vi "TemperatureControl_CuiLab.vi"() -> ()   [LabVIEW 2017]
uses:
  <vilib>/Utility/file.llb/Write To Spreadsheet File (string).vi
  <instrlib>/Lake Shore 335/Public/Data/Sensor Data (Single Reading).vi
  <vilib>/Analysis/NI_AALPro.lvlib
panel:
  in  "Interval":dbl=5.0 caption="Every" format="%#_g s"
  in  "TimeStamp":dbl[](array[numeric])
  in  "T history":dbl[][](array[numeric])
  in  "Set PID":bool
  in  "Sample Temp":enum16{"A", "B", "C", "D"}(ring)
  in  "Write to File":bool
  in  "Interval (ms)":i32=500
  in  "Temperature Log File":path
  out "Temperature":T1(graph)
  out "Temp D":dbl=11.245 caption="D:"
  out "Temp C":dbl=4.276 caption="C:"
  out "Standalone":bool=TRUE
  in  "Set":bool
  in  "Refresh":bool
  in  "Manual Output (%)":dbl
  in  "Loop 1 Heater Range":u16(ring)=3 items=["Off", "Low (0.5W)", "Med (5W)", "High (50W)"]
  in  "Rate (D)":dbl=20.0
  in  "Reset (I)":dbl=10.0
  in  "Gain (P)":dbl=10.0
  in  "Ramp Rate (K/min)":dbl=10.0
  in  "Ramp":bool=TRUE
  in  "Setpoint (K)":dbl=4.0
  in  "Quit":bool
  in  "Loop":u16(ring) items=["1"=1, "2"=2]
  in  "Model":enum16{"LS 335", "LS 340"}(ring)
  in  "VISA resource name":refnum<visa-resource-name>="Lakeshore"
  in  "Connect":bool
  out "Heater Output":dbl(slide) scale=0.0..100.0
  out "Heater Range Status":string="High"
  out "Setpoint status":dbl=4.0 caption="S:"
  out "Temp B":dbl=11.245 caption="B:"
  out "Temp A":dbl=4.276 caption="A:"
  # "Rates (K/min)"
  # "K"
  # "K"
  # "K"
  # "K"
  # "K"
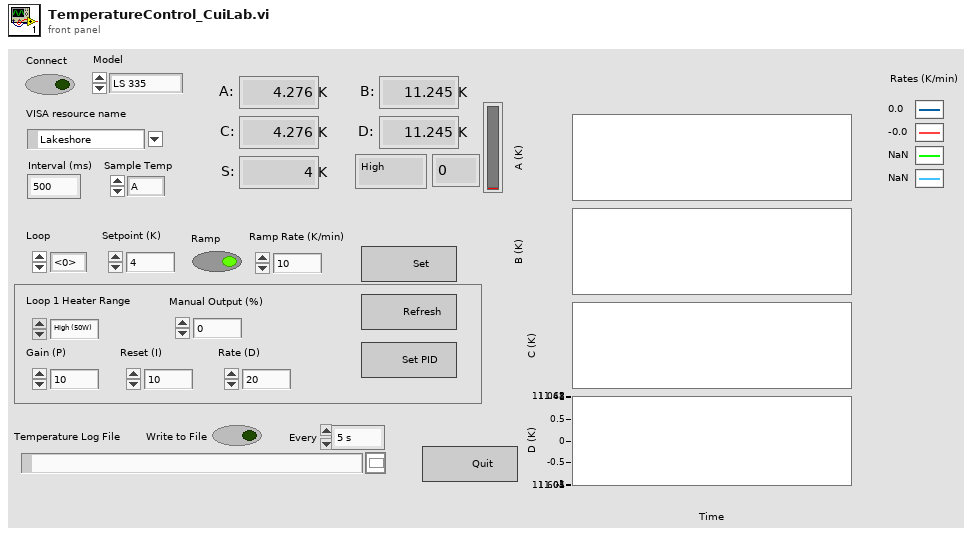
[diagram p1: front panel]
types:
  T1 = cluster{"[0]":dbl, "[1]":dbl, "[2]":dbl, "[3]":dbl}
  T2 = enum16{"Init", "Read", "ScannerVXY", "ScannerVZ", "ScannerVXYZ", "Temp", "Field", "He", "Encoder", "MIM", "NanonisMon", "ScannerXYZ"}
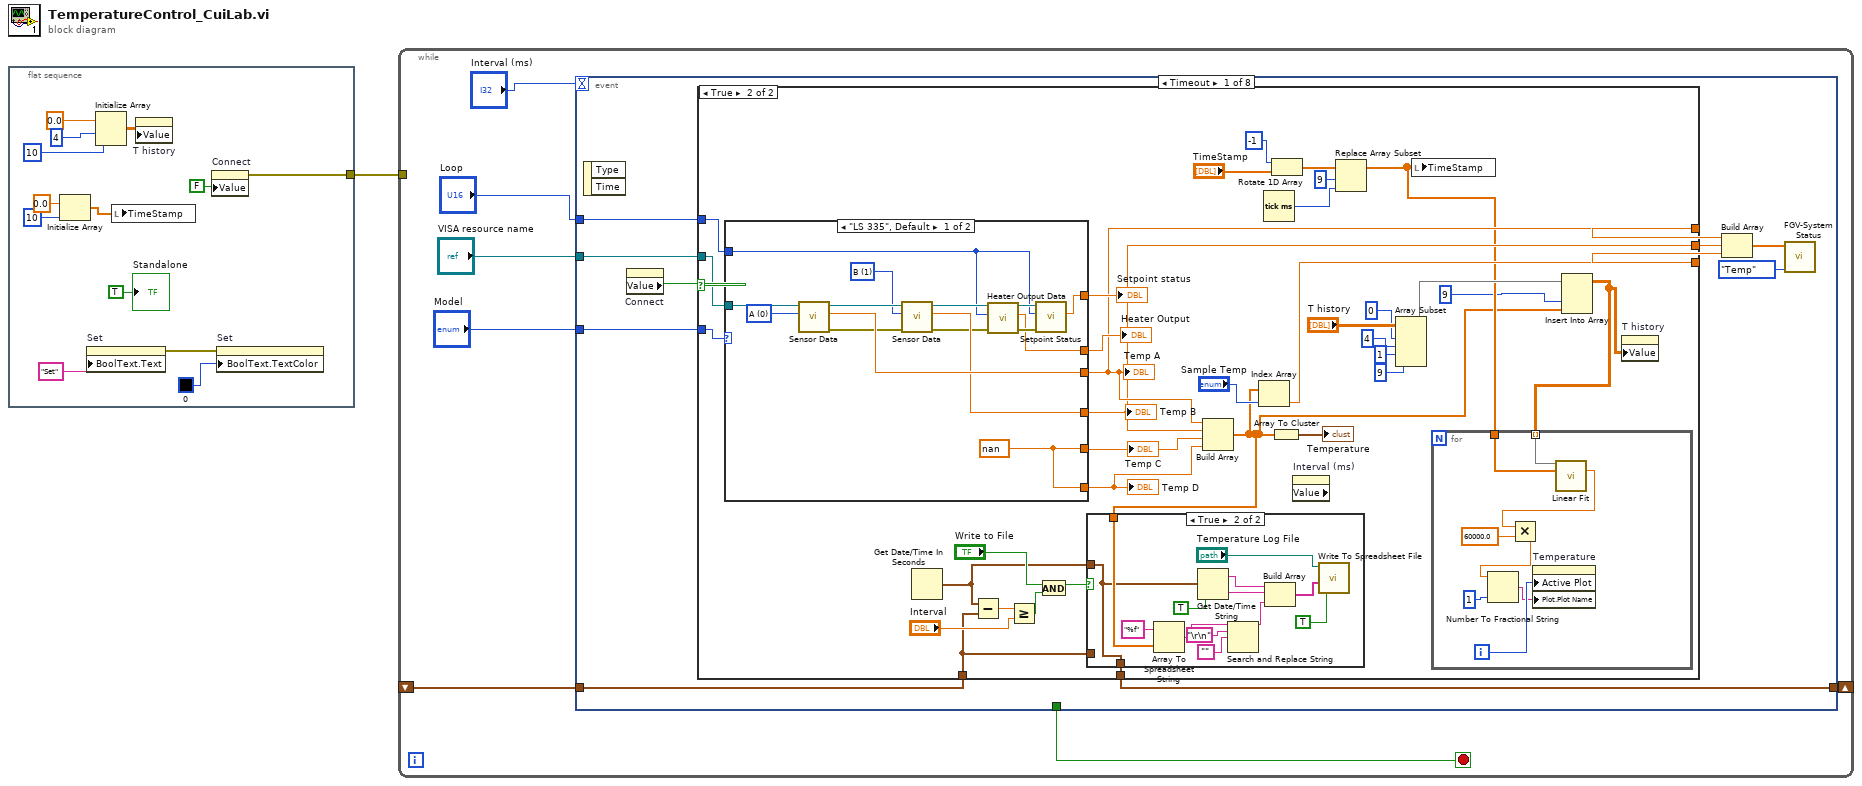
[diagram p0: block diagram]
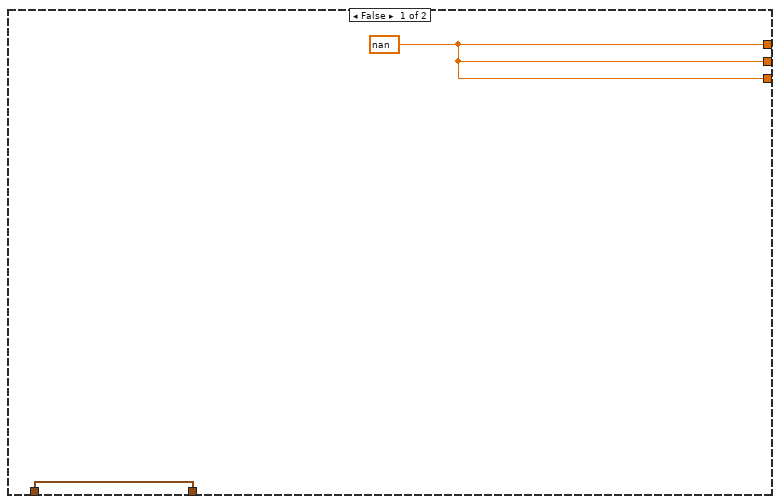
[diagram p2: hidden frame]
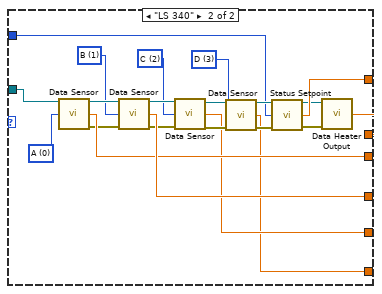
[diagram p4: hidden frame]
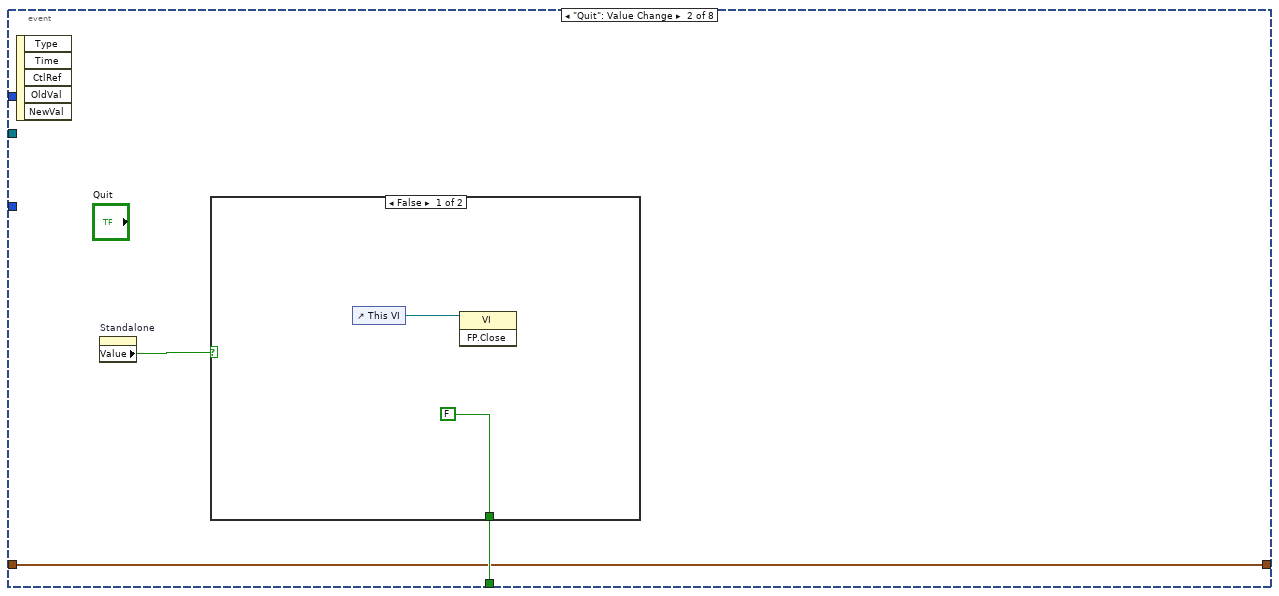
[diagram p5: hidden frame]
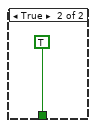
[diagram p6: hidden frame]
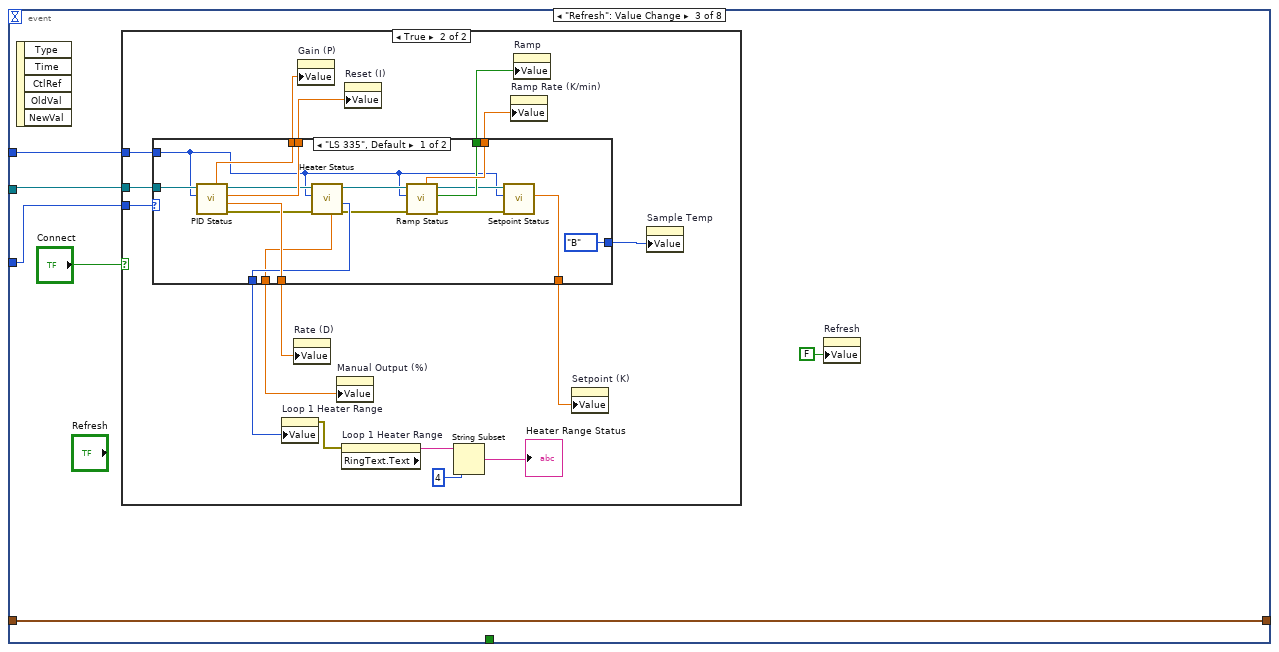
[diagram p7: hidden frame]
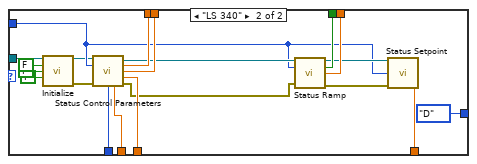
[diagram p9: hidden frame]
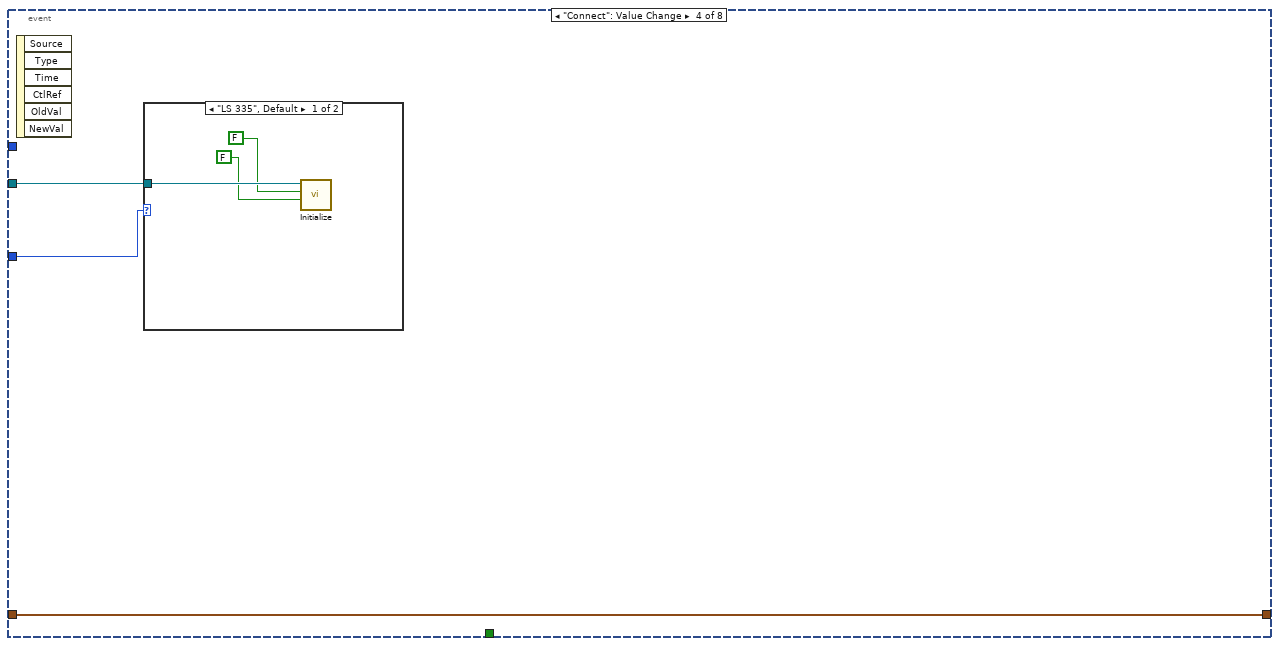
[diagram p10: hidden frame]
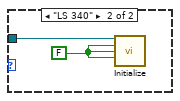
[diagram p11: hidden frame]
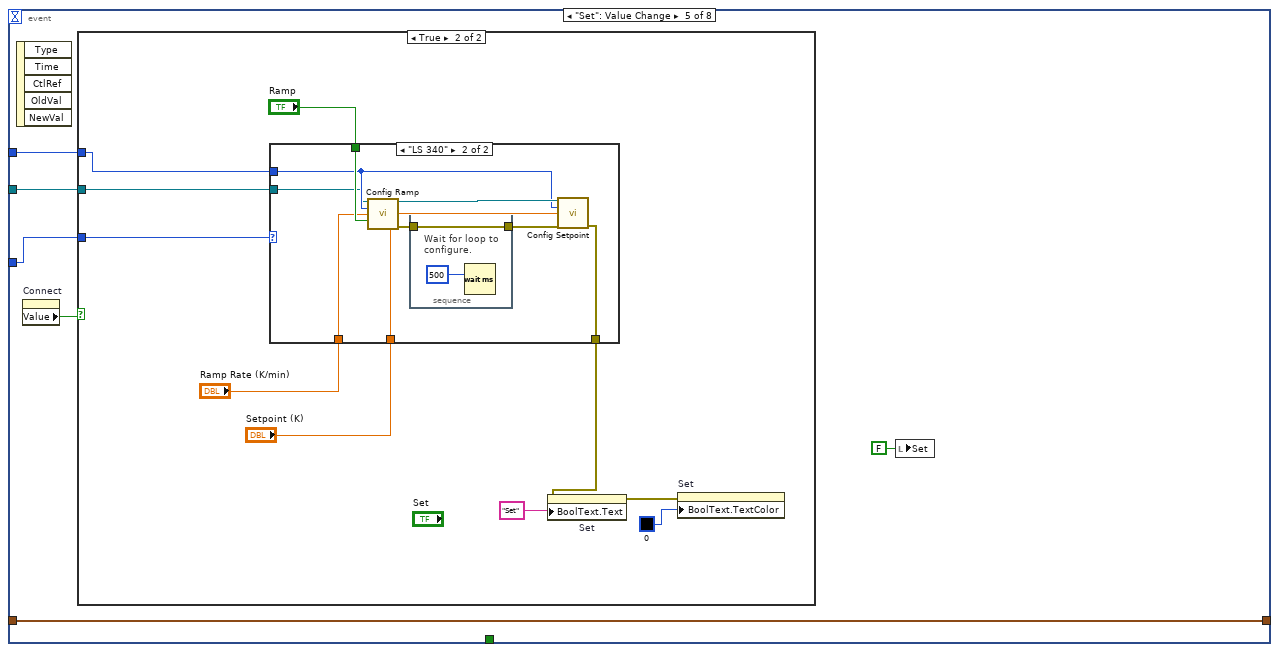
[diagram p12: hidden frame]
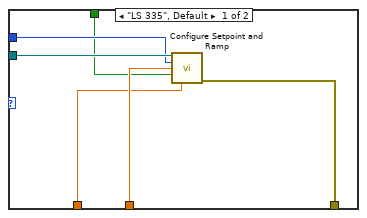
[diagram p14: hidden frame]
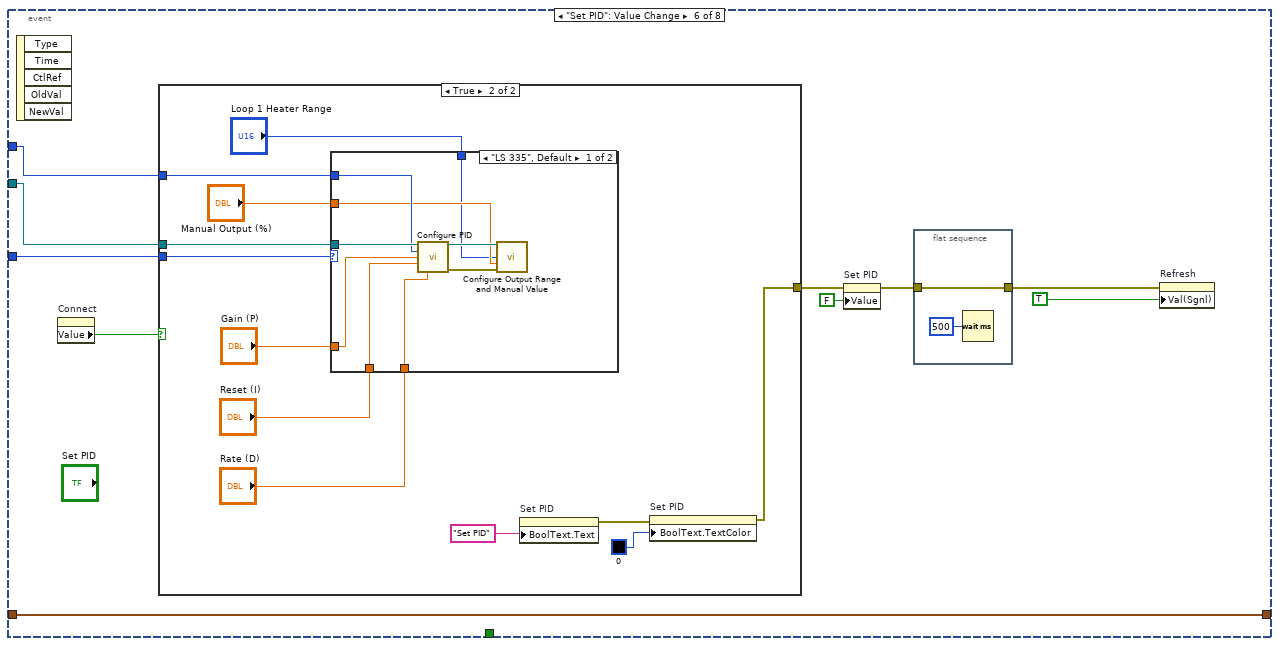
[diagram p15: hidden frame]
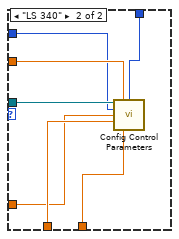
[diagram p17: hidden frame]
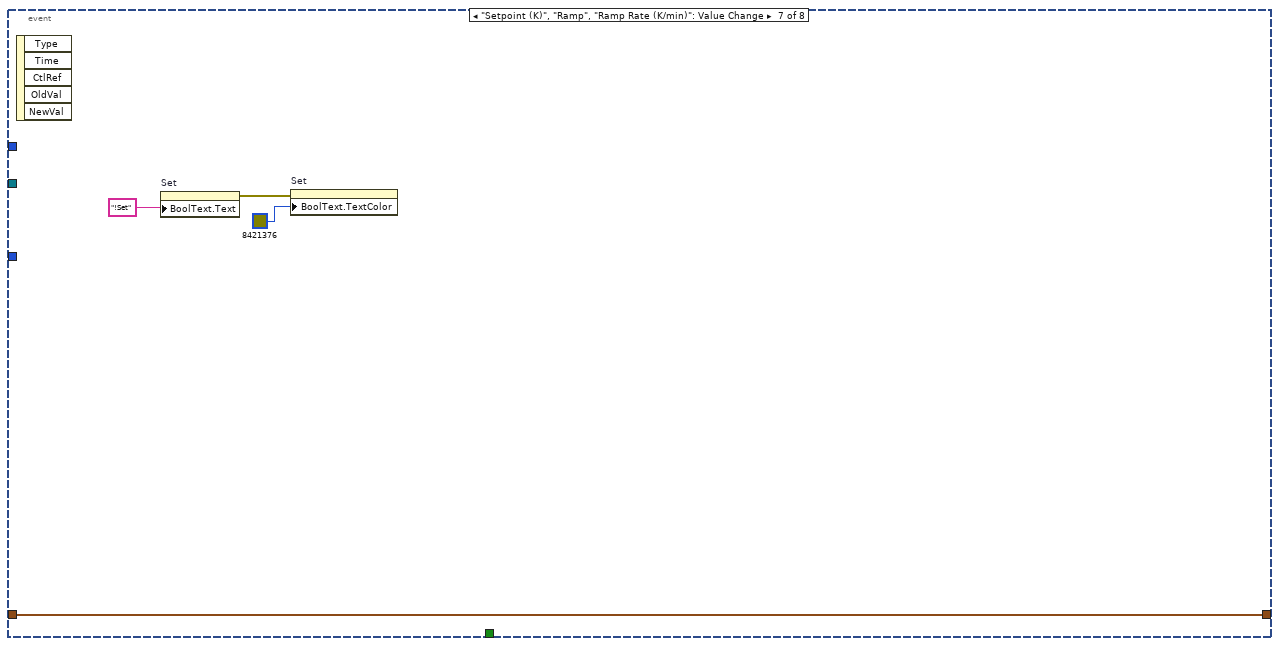
[diagram p18: hidden frame]
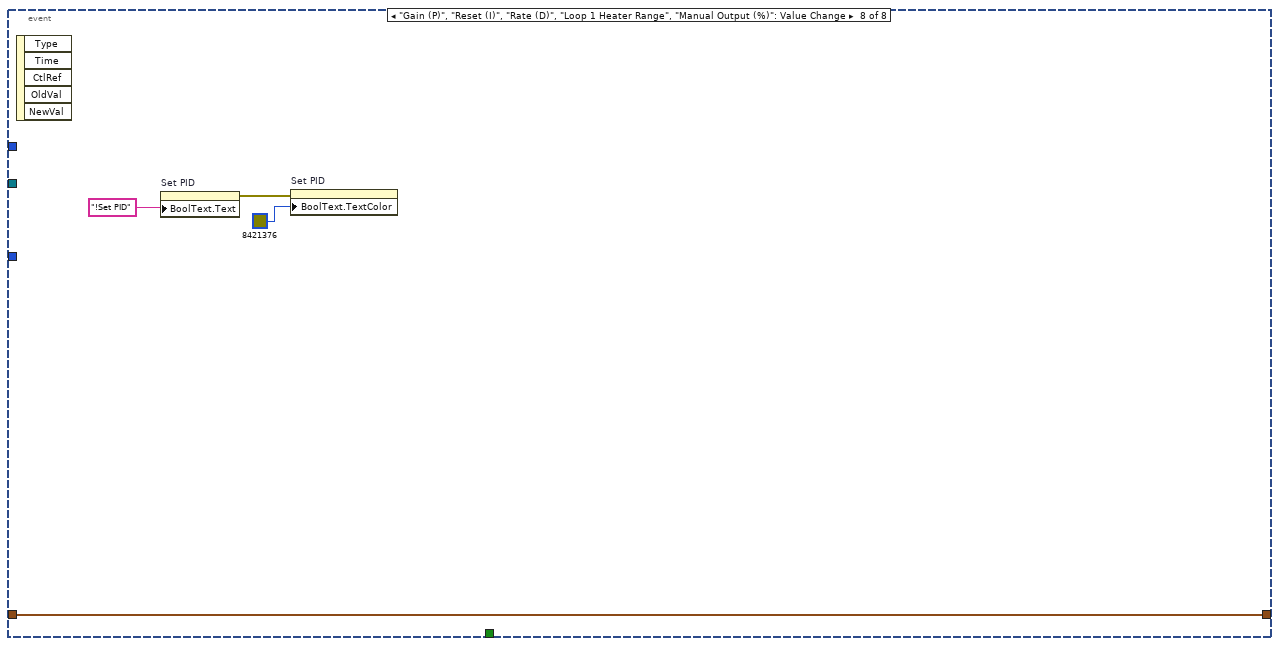
[diagram p19: hidden frame]
diagram:
  n1 = flat-sequence {
    tunnel: [w13] -> w1
    frame #0 {
      n2 = Initialize Array(0.0 ("element"), 10 ("dimension size")) -> (w2:dbl[])
      n3 = property on="Set" class="Bool (strict)"("BoolText.Text"="Set" ("Label.Text")) -> (error out=w10:errorcluster)  [unwired: 2 in, 1 out]
      n4 = Initialize Array(0.0 ("element"), 4 ("dimension size"), 10 ("dimension size")) -> (w6:dbl[][])
      n5 = local write "TimeStamp"(w2) -> ()
      n6 = property on="T history" class="Arr (strict)"("Value"=w6) -> ()  [unwired: 2 in, 2 out]
      n7 = property on="Connect" class="Bool (strict)"("Value"=FALSE ("Connect")) -> (error out=w13:errorcluster)  [unwired: 2 in, 1 out]
      n8 = property on="Set" class="Bool (strict)"(error in=w10, "BoolText.TextColor"=u32 0) -> ()  [unwired: 1 in, 2 out]
      "Standalone" <- TRUE ("Standalone")
    }
  }
  n9 = while {
    tunnel: w1 -> [_]
    shift-right: [w16] -> _
    shift-left: _ -> [w15]
    stop <- w18 stop-if-true
    n10 = event shown="[0] Timeout" {
      selector: _ -> [_ _ _ _ _ _ _ _]
      dyn-events: _ -> [_ _ _ _ _ _ _ _]
      timeout: "Interval (ms)" -> [_ _ _ _ _ _ _ _]
      tunnel: "VISA resource name" -> [w32 _ w140 w196 w207 w242 _ _]
      tunnel: "Model" -> [w31 _ w138 w195 w205 w243 _ _]
      tunnel: "Loop" -> [w30 _ w139 _ w206 w241 _ _]
      tunnel: [_ w130 _ _ _ _ _ _] -> w18
      tunnel: [w23 w129 w135 w194 w202 w235 w275 w279] -> w16
      tunnel: w15 -> [w22 w129 w135 w194 w202 w235 w275 w279]
      event Timeout {
        n11 = event-data() -> ()  [unwired: 1 in, 2 out]
        n12 = property on="Connect" class="Bool (strict)"() -> ("Value"=w29:bool)  [unwired: 2 in, 2 out]
        n13 = case shown="True" w29 {
          tunnel: w32 -> [_ w69]
          tunnel: w31 -> [_ w68]
          tunnel: w30 -> [_ w67]
          tunnel: [w34 w59] -> w28
          tunnel: [w34 w58] -> w27
          tunnel: [w34 w57] -> w26
          tunnel: [w33 w44] -> w23
          tunnel: w22 -> [w33 w38]
          frame False {
            w34 = nan ("Kelvin Reading")
          }
          frame True {
            n14 = case shown="\"LS 335\", Default" w68 {
              tunnel: w69 -> [w105 w128]
              tunnel: [w103 w123] -> w59
              tunnel: [w100 w124] -> w58
              tunnel: [w96 w122] -> w66
              tunnel: [w92 w119] -> w65
              tunnel: [w106 w109] -> w62
              tunnel: [w106 w108] -> w61
              tunnel: w67 -> [w94 w107]
              frame "LS 335", Default {
                w101 = u16 1 items=["A", "B"] ("Input (0:A)")
                w104 = u16 0 items=["A", "B"] ("Input (0:A)")
                w106 = nan ("Kelvin Reading")
                n15 = call-poly <instrlib>:"Sensor Data.vi"("Input (0:A)"=w104, "VISA resource name"=w105) -> ("error out"=w98:errorcluster, "Sensor Data"=w103:dbl, "VISA resource name out"=w102:refnum<visa-resource-name>)  [unwired: 7 in]
                n16 = call-poly <instrlib>:"Sensor Data.vi"("error in (no error)"=w98, "Input (0:A)"=w101, "VISA resource name"=w102) -> ("error out"=w97:errorcluster, "Sensor Data"=w100:dbl, "VISA resource name out"=w99:refnum<visa-resource-name>)  [unwired: 6 in]
                n17 = call <instrlib>:"Heater Output Data.vi"("error in (no error)"=w97, "Heater Output (1:1)"=w94, "VISA resource name"=w99) -> ("error out"=w93:errorcluster, "Output Value"=w92:dbl, "VISA resource name out"=w95:refnum<visa-resource-name>)  [unwired: 6 in]
                n18 = call <instrlib>:"Setpoint Status.vi"("error in (no error)"=w93, "Output (1:1)"=w94, "VISA resource name"=w95) -> ("Setpoint"=w96:dbl)  [unwired: 6 in, 2 out]
              }
              frame "LS 340" {
                w110 = u16 3 items=["A", "B", "C", "D"] ("Input (0: A)")
                w111 = u16 2 items=["A", "B", "C", "D"] ("Input (0: A)")
                w125 = u16 1 items=["A", "B", "C", "D"] ("Input (0: A)")
                w127 = u16 0 items=["A", "B", "C", "D"] ("Input (0: A)")
                n19 = call <instrlib>:"Data Sensor.vi"("VISA resource name"=w128, "Input (0: A)"=w127) -> ("VISA resource name out"=w126:refnum<visa-resource-name>, "Kelvin Reading"=w123:dbl, "error out"=w118:errorcluster)  [unwired: 9 in, 2 out]
                n20 = call <instrlib>:"Data Sensor.vi"("VISA resource name"=w126, "Input (0: A)"=w125, "error in (no error)"=w118) -> ("VISA resource name out"=w117:refnum<visa-resource-name>, "Kelvin Reading"=w124:dbl, "error out"=w116:errorcluster)  [unwired: 8 in, 2 out]
                n21 = call <instrlib>:"Data Sensor.vi"("VISA resource name"=w117, "Input (0: A)"=w111, "error in (no error)"=w116) -> ("VISA resource name out"=w115:refnum<visa-resource-name>, "Kelvin Reading"=w109:dbl, "error out"=w112:errorcluster)  [unwired: 8 in, 2 out]
                n22 = call <instrlib>:"Data Sensor.vi"("VISA resource name"=w115, "Input (0: A)"=w110, "error in (no error)"=w112) -> ("VISA resource name out"=w114:refnum<visa-resource-name>, "Kelvin Reading"=w108:dbl, "error out"=w113:errorcluster)  [unwired: 8 in, 2 out]
                n23 = call <instrlib>:"Status Setpoint.vi"("VISA resource name"=w114, "Loop (0: 1)"=w107, "error in (no error)"=w113) -> ("VISA resource name out"=w121:refnum<visa-resource-name>, "Setpoint"=w122:dbl, "error out"=w120:errorcluster)  [unwired: 10 in]
                n24 = call <instrlib>:"Data Heater Output.vi"("VISA resource name"=w121, "error in (no error)"=w120) -> ("Heater Output"=w119:dbl)  [unwired: 11 in, 2 out]
              }
            }
            "Temp A" <- w59
            "Temp B" <- w58
            "Setpoint status" <- w66
            "Heater Output" <- w65
            "Temp D" <- w61
            "Temp C" <- w62
            n25 = Get Date/Time In Seconds() -> (seconds since 1Jan1904=w43:timestamp)
            n26 = Subtract(x=w43, y=w38) -> (x-y=w42:dbl)
            n27 = Greater Or Equal?(x=w42, y="Interval") -> (x >= y?=w39:bool)
            n28 = And(x="Write to File", y=w39) -> (x .and. y?=w40:bool)
            n29 = Build Array(w59, w58, w62, w61) -> (w37:dbl[])
            n30 = case shown="True" w40 {
              tunnel: w37 -> [_ w84]
              tunnel: [w78 w79] -> w44
              tunnel: w43 -> [_ w79]
              tunnel: w38 -> [w78 _]
              frame False {
              }
              frame True {
                n31 = Array To Spreadsheet String(array=w84, 3:"%f" ("format string")) -> (spreadsheet string=w82:string)  [unwired: 1 in]
                n32 = Get Date/Time String(seconds (now)=w79, want seconds? (F)=TRUE) -> (date string=w90:string, time string=w89:string)  [unwired: 1 in]
                n33 = Search and Replace String(input string=w82, search string="\r\n", replace string="") -> (result string=w83:string)  [unwired: 5 in, 3 out]
                n34 = Build Array(w90, w89, w83) -> (w87:string[])
                n35 = call-poly <vilib>:"Write To Spreadsheet File.vi"("append to file? (new file:F)"=TRUE, "1D data"=w87, "file path (dialog if empty)"="Temperature Log File") -> ()  [unwired: 5 in, 1 out]
              }
            }
            n36 = Index Array(array=w37, index="Sample Temp") -> (element=w57:dbl)
            n37 = Tick Count (ms)() -> (millisecond timer value=w46:u32)
            n38 = Array To Cluster(array=w37) -> (cluster=→"Temperature":T1)
            n39 = Rotate 1D Array(1:"TimeStamp", 2:-1 ("n")) -> (0:w48:dbl[])
            n40 = property on="Interval (ms)" class="DigNum (strict)" props=["Value"]() -> ()  [unwired: 2 in, 3 out]
            n41 = Replace Array Subset(array=w48, new element=w46, index=9) -> (w45:dbl[])
            n42 = Array Subset(array="T history", index (row)=0 ("index"), length (row)=4 ("length"), index (col)=1 ("index"), length (col)=9 ("length")) -> (w51:dbl[][])
            n43 = local write "TimeStamp"(w45) -> ()
            n44 = Insert Into Array(array=w51, index (col)=9 ("disabled index (col)"), new element=w37) -> (w36:dbl[][])  [unwired: 1 in]
            n45 = for {
              tunnel: w45 -> [w73]
              tunnel: w36 -> [w70] mode=indexing
              i -> [w77]
              n46 = call <vilib>:"Linear Fit.vi"("Y"=w70, "X"=w73) -> ("slope"=w71:dbl)  [unwired: 9 in, 4 out]
              n47 = Multiply(x=w71, y=60000.0) -> (x*y=w76:dbl)
              n48 = Number To Fractional String(number=w76, precision (6)=i16 1) -> (F-format string=w74:string)  [unwired: 2 in]
              n49 = property on="Temperature" class="WFChart (strict)"("Active Plot"=w77, "Plot.Plot Name"=w74) -> ()  [unwired: 2 in, 2 out]
            }
            n50 = property on="T history" class="Arr (strict)"("Value"=w36) -> ()  [unwired: 2 in, 2 out]
          }
        }
        n51 = Build Array(w28, w27, w26) -> (w25:dbl[])
        n52 = call "FGV-System Status.vi"("Action"=T2."Temp", "Input Data"=w25) -> ()  [unwired: 9 in, 1 out]
      }
      event "Quit": Value Change {
        n53 = event-data() -> ()  [unwired: 1 in, 5 out]
        n54 = property on="Standalone" class="Bool (strict)"() -> ("Value"=w131:bool)  [unwired: 2 in, 2 out]
        n55 = case shown="False" w131 {
          tunnel: [FALSE TRUE] -> w130
          frame False {
            n56 = control-ref of="This VI"() -> (w132:refnum<vi>)
            n57 = invoke class="VI" method="FP.Close"(reference=w132) -> ()  [unwired: 2 in, 3 out]
          }
          frame True {
          }
        }
      }
      event "Refresh": Value Change {
        n58 = event-data() -> ()  [unwired: 1 in, 5 out]
        n59 = case shown="True" "Connect" {
          tunnel: w140 -> [_ w156]
          tunnel: w139 -> [_ w149]
          tunnel: w138 -> [_ w146]
          frame False {
          }
          frame True {
            n60 = case shown="\"LS 335\", Default" w146 {
              tunnel: w156 -> [w172 w178]
              tunnel: [w170 w193] -> w155
              tunnel: [w171 w192] -> w154
              tunnel: [w169 w191] -> w153
              tunnel: [w166 w190] -> w152
              tunnel: [w162 w187] -> w151
              tunnel: [w163 w186] -> w150
              tunnel: w149 -> [w159 w183]
              tunnel: [w157 w182] -> w148
              tunnel: [w167 w181] -> w147
              tunnel: [enum16{"A", "B", "C", "D"}."B" ("Sample Temp") enum16{"A", "B", "C", "D"}."D" ("Sample Temp")] -> w141
              frame "LS 335", Default {
                n61 = call <instrlib>:"PID Status.vi"("Output's Control Loop (1:1)"=w159, "VISA resource name"=w172) -> ("error out"=w165:errorcluster, "Rate (D)"=w169:dbl, "Reset (I)"=w171:dbl, "VISA resource name out"=w168:refnum<visa-resource-name>, "Gain (P)"=w170:dbl)  [unwired: 5 in]
                n62 = call <instrlib>:"Heater Status.vi"("error in (no error)"=w165, "Heater Output (1:1)"=w159, "VISA resource name"=w168) -> ("error out"=w161:errorcluster, "Heater Range"=w167:u16, "VISA resource name out"=w164:refnum<visa-resource-name>, "Manual Output Value"=w166:dbl)  [unwired: 4 in, 1 out]
                n63 = call <instrlib>:"Ramp Status.vi"("error in (no error)"=w161, "Output's Control Loop (1:1)"=w159, "VISA resource name"=w164) -> ("error out"=w158:errorcluster, "Ramping On"=w162:bool, "VISA resource name out"=w160:refnum<visa-resource-name>, "Ramp Rate"=w163:dbl)  [unwired: 4 in, 1 out]
                n64 = call <instrlib>:"Setpoint Status.vi"("error in (no error)"=w158, "Output (1:1)"=w159, "VISA resource name"=w160) -> ("Setpoint"=w157:dbl)  [unwired: 6 in, 2 out]
              }
              frame "LS 340" {
                n65 = call <instrlib>:"Initialize.vi"("VISA resource name"=w178, "ID Query (T: Check)"=FALSE, "Reset (T: Reset)"=FALSE, "Reset Defaults (F:Dont Reset)"=FALSE) -> ("VISA resource name out"=w180:refnum<visa-resource-name>, "error out"=w179:errorcluster)  [unwired: 10 in]
                n66 = call <instrlib>:"Status Control Parameters.vi"("VISA resource name"=w180, "Loop (0: 1)"=w183, "error in (no error)"=w179) -> ("VISA resource name out"=w189:refnum<visa-resource-name>, "Gain (P)"=w193:dbl, "Reset (I)"=w192:dbl, "Rate (D)"=w191:dbl, "Loop 1 Heater Range"=w181:u16, "Manual Output"=w190:dbl, "error out"=w188:errorcluster)  [unwired: 5 in, 1 out]
                n67 = call <instrlib>:"Status Ramp.vi"("VISA resource name"=w189, "Loop (0: 1)"=w183, "error in (no error)"=w188) -> ("VISA resource name out"=w185:refnum<visa-resource-name>, "Ramping On/Off"=w187:bool, "Rate Value"=w186:dbl, "error out"=w184:errorcluster)  [unwired: 8 in, 1 out]
                n68 = call <instrlib>:"Status Setpoint.vi"("VISA resource name"=w185, "Loop (0: 1)"=w183, "error in (no error)"=w184) -> ("Setpoint"=w182:dbl)  [unwired: 10 in, 2 out]
              }
            }
            n69 = property on="Loop 1 Heater Range" class="Ring (strict)"("Value"=w147) -> (error out=w145:errorcluster)  [unwired: 2 in, 1 out]
            n70 = property on="Rate (D)" class="DigNum (strict)"("Value"=w153) -> ()  [unwired: 2 in, 2 out]
            n71 = property on="Gain (P)" class="DigNum (strict)"("Value"=w155) -> ()  [unwired: 2 in, 2 out]
            n72 = property on="Manual Output (%)" class="DigNum (strict)"("Value"=w152) -> ()  [unwired: 2 in, 2 out]
            n73 = property on="Loop 1 Heater Range" class="Ring (strict)"(error in=w145) -> ("RingText.Text"=w144:string)  [unwired: 1 in, 2 out]
            n74 = property on="Reset (I)" class="DigNum (strict)"("Value"=w154) -> ()  [unwired: 2 in, 2 out]
            n75 = String Subset(string=w144, length (rest)=4 ("length (rest)")) -> (substring=→"Heater Range Status":string)  [unwired: 1 in]
            n76 = property on="Ramp Rate (K/min)" class="DigNum (strict)"("Value"=w150) -> ()  [unwired: 2 in, 2 out]
            n77 = property on="Ramp" class="Bool (strict)"("Value"=w151) -> ()  [unwired: 2 in, 2 out]
            n78 = property on="Setpoint (K)" class="DigNum (strict)"("Value"=w148) -> ()  [unwired: 2 in, 2 out]
            n79 = property on="Sample Temp" class="Enum (strict)"("Value"=w141) -> ()  [unwired: 2 in, 2 out]
          }
        }
        n80 = property on="Refresh" class="Bool (strict)"("Value"=FALSE ("Refresh")) -> ()  [unwired: 2 in, 2 out]
      }
      event "Connect": Value Change {
        n81 = event-data() -> ()  [unwired: 1 in, 6 out]
        n82 = case shown="\"LS 335\", Default" w195 {
          tunnel: w196 -> [w199 w201]
          frame "LS 335", Default {
            n83 = call <instrlib>:"Initialize.vi"("Reset (True)"=FALSE ("ID Query (True)"), "ID Query (True)"=FALSE ("Reset (True)"), "VISA resource name"=w199) -> ()  [unwired: 7 in, 2 out]
          }
          frame "LS 340" {
            w200 = FALSE ("ID Query (T: Check)")
            n84 = call <instrlib>:"Initialize.vi"("VISA resource name"=w201, "ID Query (T: Check)"=w200, "Reset (T: Reset)"=w200, "Reset Defaults (F:Dont Reset)"=w200) -> ()  [unwired: 10 in, 2 out]
          }
        }
      }
      event "Set": Value Change {
        n85 = event-data() -> ()  [unwired: 1 in, 5 out]
        n86 = property on="Connect" class="Bool (strict)"() -> ("Value"=w204:bool)  [unwired: 2 in, 2 out]
        n87 = case shown="True" w204 {
          tunnel: w207 -> [_ w210]
          tunnel: w206 -> [_ w209]
          tunnel: w205 -> [_ w208]
          frame False {
          }
          frame True {
            n88 = case shown="\"LS 340\"" w208 {
              tunnel: w210 -> [w223 w224]
              tunnel: "Ramp" -> [w220 w232]
              tunnel: "Ramp Rate (K/min)" -> [w219 w231]
              tunnel: "Setpoint (K)" -> [w221 w229]
              tunnel: [w218 w226] -> w211
              tunnel: w209 -> [w222 w225]
              frame "LS 335", Default {
                n89 = call <instrlib>:"Configure Setpoint and Ramp.vi"("VISA resource name"=w223, "Output's Control Loop (1:1)"=w222, "Setpoint (0.0000)"=w221, "Enable Setpoint Ramping (F: Off)"=w220, "Ramp Rate (0.0)"=w219) -> ("error out"=w218:errorcluster)  [unwired: 9 in, 1 out]
              }
              frame "LS 340" {
                n90 = call <instrlib>:"Config Ramp.vi"("VISA resource name"=w224, "Loop (0: 1)"=w225, "Rate Value (0.1)"=w231, "Ramping On/Off (F: Ramping Off)"=w232) -> ("VISA resource name out"=w230:refnum<visa-resource-name>, "error out"=w228:errorcluster)  [unwired: 10 in]
                n91 = stacked-sequence {
                  tunnel: w228 -> [w233]
                  tunnel: [w233] -> w227
                  frame #0 {
                    # "Wait for loop to \nconfigure."
                    n92 = Wait (ms)(milliseconds to wait=u32 500) -> ()  [unwired: 1 out]
                  }
                }
                n93 = call <instrlib>:"Config Setpoint.vi"("VISA resource name"=w230, "Loop (0: 1)"=w225, "Setpoint (0.0)"=w229, "error in (no error)"=w227) -> ("error out"=w226:errorcluster)  [unwired: 10 in, 1 out]
              }
            }
            n94 = property on="Set" class="Bool (strict)"(error in=w211, "BoolText.Text"="Set" ("Label.Text")) -> (error out=w213:errorcluster)  [unwired: 1 in, 1 out]
            n95 = property on="Set" class="Bool (strict)"(error in=w213, "BoolText.TextColor"=u32 0) -> ()  [unwired: 1 in, 2 out]
          }
        }
        n96 = local write "Set"(FALSE ("Set")) -> ()
      }
      event "Set PID": Value Change {
        n97 = event-data() -> ()  [unwired: 1 in, 5 out]
        n98 = property on="Connect" class="Bool (strict)"() -> ("Value"=w244:bool)  [unwired: 2 in, 2 out]
        n99 = case shown="True" w244 {
          tunnel: w243 -> [_ w258]
          tunnel: w242 -> [_ w257]
          tunnel: w241 -> [_ w256]
          tunnel: [_ w247] -> w238
          frame False {
          }
          frame True {
            n100 = case shown="\"LS 335\", Default" w258 {
              tunnel: w257 -> [w267 w274]
              tunnel: w256 -> [w263 w271]
              tunnel: "Loop 1 Heater Range" -> [w259 w273]
              tunnel: "Manual Output (%)" -> [w260 w272]
              tunnel: "Reset (I)" -> [w264 w269]
              tunnel: "Rate (D)" -> [w262 w270]
              tunnel: "Gain (P)" -> [w265 w268]
              frame "LS 335", Default {
                n101 = call <instrlib>:"Configure PID.vi"("VISA resource name"=w267, "Output's Control Loop (1:1)"=w263, "Gain (P) (50.0)"=w265, "Reset (I) (20.0)"=w264, "Rate (D) (0.0 %)"=w262) -> ("VISA resource name out"=w266:refnum<visa-resource-name>, "error out"=w261:errorcluster)  [unwired: 9 in]
                n102 = call <instrlib>:"Configure Output Range and Manual Value.vi"("VISA resource name"=w266, "Range (0:Off)"=w259, "Manual Output (0.00 %)"=w260, "error in (no error)"=w261) -> ()  [unwired: 10 in, 2 out]
              }
              frame "LS 340" {
                n103 = call <instrlib>:"Config Control Parameters.vi"("VISA resource name"=w274, "Manual Output (0.00)"=w272, "Heater Range (0: Off)"=w273, "Loop (0: 1)"=w271, "Gain (P) (0.0)"=w268, "Reset (I) (0.0)"=w269, "Rate (D) (0)"=w270) -> ()  [unwired: 7 in, 2 out]
              }
            }
            n104 = property on="Set PID" class="Bool (strict)"("BoolText.Text"="Set PID" ("Label.Text")) -> (error out=w249:errorcluster)  [unwired: 2 in, 1 out]
            n105 = property on="Set PID" class="Bool (strict)"(error in=w249, "BoolText.TextColor"=u32 0) -> (error out=w247:errorcluster)  [unwired: 1 in, 1 out]
          }
        }
        n106 = property on="Set PID" class="Bool (strict)"(error in=w238, "Value"=FALSE ("Set PID")) -> (error out=w237:errorcluster)  [unwired: 1 in, 1 out]
        n107 = flat-sequence {
          tunnel: w237 -> [w245]
          tunnel: [w245] -> w236
          frame #0 {
            n108 = Wait (ms)(milliseconds to wait=u32 500) -> ()  [unwired: 1 out]
          }
        }
        n109 = property on="Refresh" class="Bool (strict)"(error in=w236, "Val(Sgnl)"=TRUE ("Value (Signaling)")) -> ()  [unwired: 1 in, 2 out]
      }
      event "Setpoint (K)", "Ramp", "Ramp Rate (K/min)": Value Change {
        n110 = event-data() -> ()  [unwired: 1 in, 5 out]
        n111 = property on="Set" class="Bool (strict)"("BoolText.Text"="!Set" ("Label.Text")) -> (error out=w277:errorcluster)  [unwired: 2 in, 1 out]
        n112 = property on="Set" class="Bool (strict)"(error in=w277, "BoolText.TextColor"=u32 8421376) -> ()  [unwired: 1 in, 2 out]
      }
      event "Gain (P)", "Reset (I)", "Rate (D)", "Loop 1 Heater Range", "Manual Output (%)": Value Change {
        n113 = event-data() -> ()  [unwired: 1 in, 5 out]
        n114 = property on="Set PID" class="Bool (strict)"("BoolText.Text"="!Set PID" ("Label.Text")) -> (error out=w281:errorcluster)  [unwired: 2 in, 1 out]
        n115 = property on="Set PID" class="Bool (strict)"(error in=w281, "BoolText.TextColor"=u32 8421376) -> ()  [unwired: 1 in, 2 out]
      }
    }
  }
